vi "Preset.vi"(7 "Array":i16[](array[numeric]), 8 "error in (no error)":errorcluster, 9 "CT":i32, 10 "CL":i32, 11 "queue in":refnum<queue>) -> (0 "error out":errorcluster, 1 "Text CT":string, 2 "Text CL":string, 3 "queue out":refnum<queue>, 5 "output array":i16[](array[numeric]))   [LabVIEW 2023]
uses:
  usr/local/natinst/LabVIEW-2023-64/examples/Design Patterns/Queued Message Handler/support/QMH Fundamentals - Message Cluster.ctl
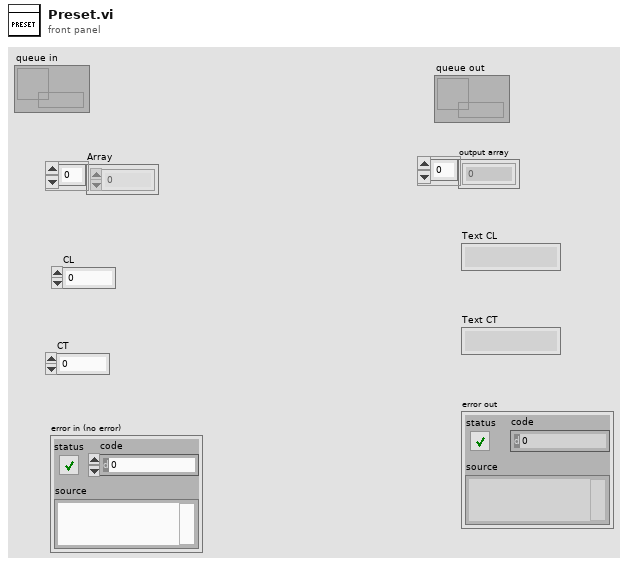
[diagram p1: front panel]
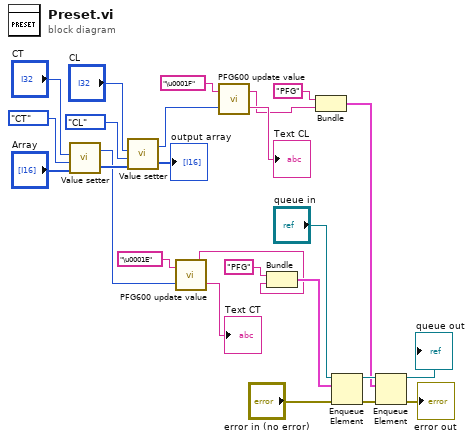
[diagram p0: block diagram]
diagram:
  n1 = call "Value setter.vi"("Array"="Array", "Enum"=enum16{"FWD", "CL", "CT", "Ar", "O2", "Timer"}."CT", "value"="CT") -> ("output array"=w20:i16[], "value"=w16:i16)  [unwired: 1 in]
  n2 = call "Value setter.vi"("Array"=w20, "Enum"=enum16{"FWD", "CL", "CT", "Ar", "O2", "Timer"}."CL", "value"="CL") -> ("output array"=→"output array":i16[], "value"=w17:i16)  [unwired: 1 in]
  n3 = call "PFG600 update value.vi"("Value"=w16, "Command"="\u0001E") -> ("Text"=→"Text CT":string, "Hex"=w1:string)
  n4 = call "PFG600 update value.vi"("Value"=w17, "Command"="\u0001F") -> ("Text"=→"Text CL":string, "Hex"=w2:string)
  n5 = Bundle("PFG", "Hex"=w1) -> (w8:cluster{string, "Hex":string})  [unwired: 1 in]
  n6 = Bundle("PFG", "Hex"=w2) -> (w4:cluster{string, "Hex":string})  [unwired: 1 in]
  n7 = Enqueue Element(queue="queue in", element=w8, error in (no error)="error in (no error)") -> (queue out=w11:refnum<queue>, error out=w23:errorcluster)  [unwired: 1 in, 1 out]
  n8 = Enqueue Element(queue=w11, element=w4, error in (no error)=w23) -> (queue out=→"queue out":refnum<queue>, error out=→"error out":errorcluster)  [unwired: 1 in, 1 out]
